vi "EX 3 1.2.vi"() -> ()   [LabVIEW 2018]
panel:
  out "Led":bool
  out "Nom":string
  out "Prénom":string
  in  "Nom brut":string
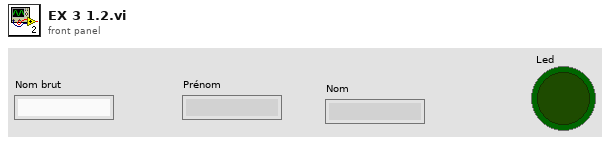
[diagram p1: front panel]
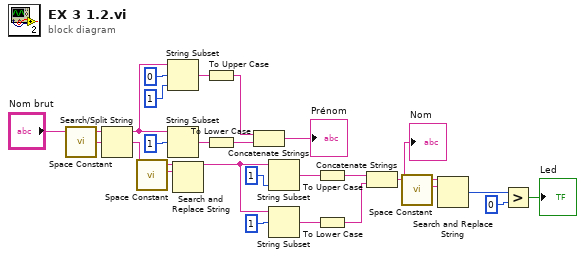
[diagram p0: block diagram]
diagram:
  n1 = call <vilib>:"Space Constant.vi"() -> ("String"=w24:string)
  n2 = Search/Split String(string="Nom brut", search string/char (-)=w24) -> (substring before match=w18:string, match + rest of string=w22:string)  [unwired: 1 in, 1 out]
  n3 = call <vilib>:"Space Constant.vi"() -> ("String"=w23:string)
  n4 = String Subset(string=w18, offset (0)=0, length (rest)=1) -> (substring=w19:string)
  n5 = String Subset(string=w18, offset (0)=1) -> (substring=w9:string)  [unwired: 1 in]
  n6 = Search and Replace String(input string=w22, search string=w23) -> (result string=w13:string)  [unwired: 6 in, 3 out]
  n7 = To Upper Case(1:w19) -> (0:w16:string)
  n8 = To Lower Case(string=w9) -> (all lower case string=w8:string)
  n9 = Concatenate Strings(w16, w8) -> (→"Prénom":string)
  n10 = String Subset(string=w13, length (rest)=1) -> (substring=w14:string)  [unwired: 1 in]
  n11 = String Subset(string=w13, offset (0)=1) -> (substring=w7:string)  [unwired: 1 in]
  n12 = To Upper Case(1:w14) -> (0:w11:string)
  n13 = To Lower Case(string=w7) -> (all lower case string=w6:string)
  n14 = Concatenate Strings(w11, w6) -> (w5:string)
  "Nom" <- w5
  n15 = call <vilib>:"Space Constant.vi"() -> ("String"=w4:string)
  n16 = Search and Replace String(input string=w5, search string=w4) -> (number of replacements=w3:i32)  [unwired: 6 in, 3 out]
  n17 = Greater?(x=w3, y=0) -> (0:→"Led":bool)
